vi "BuildBit.vi"(5 "Data Value":T3, 7 "Clock Value":T3, 9 "Number of Samples In":i32, 10 "Data Array In":u8[][](array[numeric]), 11 "RFFE_Data In":T1 {"Toggle (high to low)" items=["0", "1", "Z", "L", "H", "X", "T", "V"]; "X Array" items=["0", "1", "Z", "L", "H", "X", "T", "V"]; "Z Array" items=["0", "1", "Z", "L", "H", "X", "T", "V"]; "L Array" items=["0", "1", "Z", "L", "H", "X", "T", "V"]; "H Array" items=["0", "1", "Z", "L", "H", "X", "T", "V"]; "One Array" items=["0", "1", "Z", "L", "H", "X", "T", "V"]; "Zero Array" items=["0", "1", "Z", "L", "H", "X", "T", "V"]}) -> (1 "Number of Samples Out":i32, 2 "Data Array Out":u8[][](array[numeric]), 3 "RFFE_Data Out":T1 {"Toggle (high to low)" items=["0", "1", "Z", "L", "H", "X", "T", "V"]; "X Array" items=["0", "1", "Z", "L", "H", "X", "T", "V"]; "Z Array" items=["0", "1", "Z", "L", "H", "X", "T", "V"]; "L Array" items=["0", "1", "Z", "L", "H", "X", "T", "V"]; "H Array" items=["0", "1", "Z", "L", "H", "X", "T", "V"]; "One Array" items=["0", "1", "Z", "L", "H", "X", "T", "V"]; "Zero Array" items=["0", "1", "Z", "L", "H", "X", "T", "V"]})   [LabVIEW 2013]
doc: "This VI builds a single MIPI sample. The actual size of the same is 2x the oversample factor."
uses:
  Ctrls/RFFE_Data.ctl
  Ctrls/ClockDataChannels.ctl
  Ctrls/BitStates.ctl
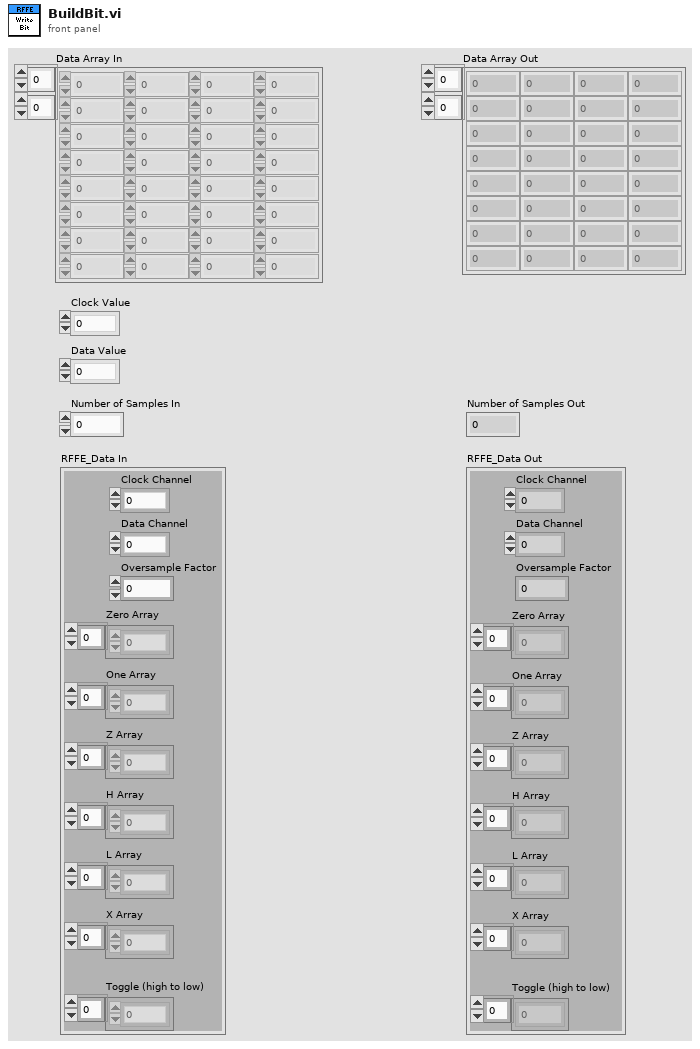
[diagram p1: front panel]
types:
  T1 = typedef "RFFE_Data.ctl" = cluster{"Clock Channel":T2, "Data Channel":T2, "Oversample Factor":u8, "Zero Array":u8[], "One Array":u8[], "Z Array ":u8[], "H Array":u8[], "L Array":u8[], "X Array":u8[], "Toggle (high to low)":u8[]}
  T2 = typedef "ClockDataChannels.ctl" = enum16{"0", "1"}
  T3 = typedef "BitStates.ctl" = enum16{"0", "1", "Z", "L", "H", "X", "Toggle"}
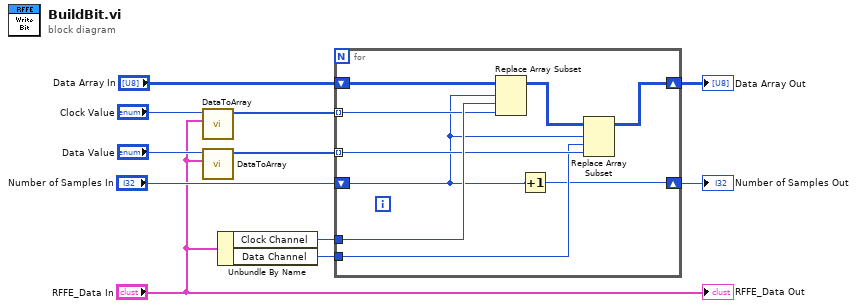
[diagram p0: block diagram]
diagram:
  n1 = call "DataToArray.vi"("RFFE_Data"="RFFE_Data In", "Value"="Clock Value") -> ("Data"=w4:u8[])  [unwired: 9 in]
  n2 = call "DataToArray.vi"("RFFE_Data"="RFFE_Data In", "Value"="Data Value") -> ("Data"=w5:u8[])  [unwired: 9 in]
  n3 = Unbundle By Name("RFFE_Data In") -> ("Clock Channel"=w8:T2, "Data Channel"=w9:T2)
  n4 = for {
    shift-right: [w17] -> w1
    shift-left: "Data Array In" -> [w20]
    tunnel: w8 -> [w19]
    tunnel: w9 -> [w14]
    tunnel: w4 -> [w18] mode=indexing
    shift-right: [w12] -> w7
    shift-left: "Number of Samples In" -> [w13]
    tunnel: w5 -> [w15] mode=indexing
    n5 = Replace Array Subset(array=w20, new element=w18, index (row)=w13, index (col)=w19) -> (w16:u8[][])
    n6 = Increment(x=w13) -> (x+1=w12:i32)
    n7 = Replace Array Subset(array=w16, new element=w15, index (row)=w13, index (col)=w14) -> (w17:u8[][])
  }
  "Data Array Out" <- w1
  "Number of Samples Out" <- w7
  "RFFE_Data Out" <- "RFFE_Data In"
